vi "NXT Obs avoid A.vi"(1 "Distance array":i16[](array[numeric])=[800, 800, 800, 800, 800, 800, 800, 800, 800, 800, 800, 800, 800, 800, 800, 800]) -> (0 "Obs array":i16[](array[numeric]))   [LabVIEW 2012, in "ENGR3390 Tug Boat.lvrbt"]
doc: "This VI creates the Obstacle Avoidance array from the scanning IR sensor. If a distance value is zero, indicating that the scan did not cover that angle, the output at that angle is set to zero. Otherwise, the output velocity is scaled from -500 to 500."
uses:
  ENGR3390 Tug Boat.lvrbt
panel:
  out "Obs array graph":i16[](graph)
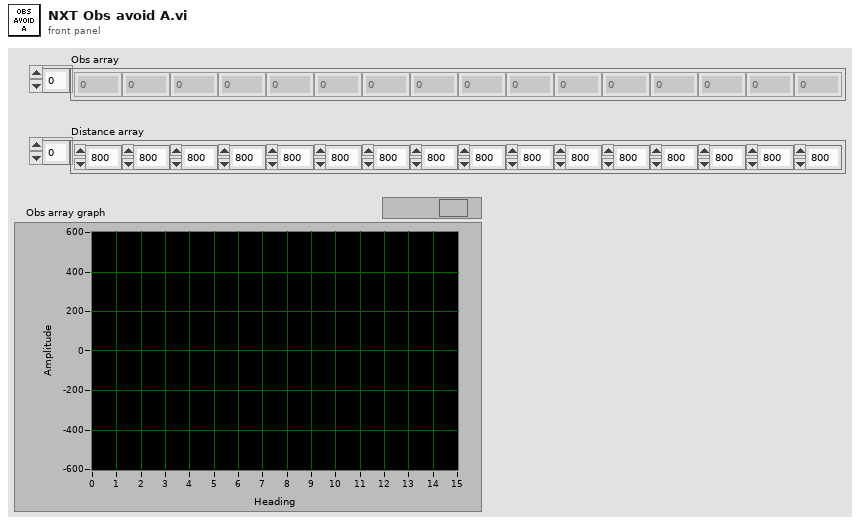
[diagram p1: front panel]
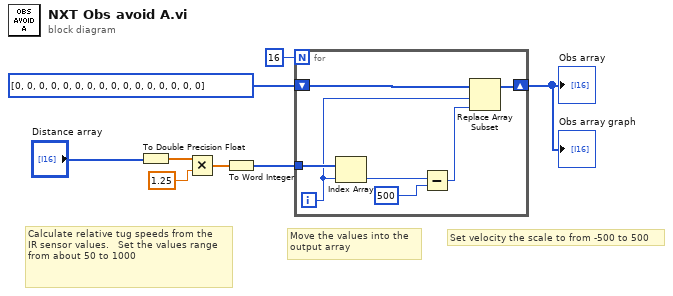
[diagram p0: block diagram]
diagram:
  # "Move the values into the\noutput array"
  # "Set velocity the scale to from -500 to 500"
  # "Calculate relative tug speeds from the\nIR sensor values.   Set the values range \nfrom about 50 to 1000"
  n1 = To Double Precision Float(number="Distance array") -> (double precision float=w8:dbl[])
  n2 = Multiply(x=w8, y=1.25) -> (x*y=w6:dbl[])
  n3 = To Word Integer(number=w6) -> (16bit integer=w2:i16[])
  n4 = for {
    N: 16 -> [_]
    tunnel: w2 -> [w15]
    shift-right: [w12] -> w1
    shift-left: i16[] [0, 0, 0, 0, 0, 0, 0, 0, 0, 0, 0, 0, 0, 0, 0, 0] ("ouput array 2") -> [w14]
    i -> [w13]
    n5 = Index Array(array=w15, index=w13) -> (element=w9:i16)
    n6 = Subtract(x=w9, y=i16 500) -> (x-y=w10:i16)
    n7 = Replace Array Subset(array=w14, new element=w10, index=w13) -> (w12:i16[])
  }
  "Obs array" <- w1
  "Obs array graph" <- w1
